vi "Image_Acquisition_Stop.vi"(11 "input cluster":T1={"L16 Linear Actuator"="ASRL6::INSTR", "XE 1000 Pump"="COM10", "Camera1"="cam2", "Camera2"="cam3", "Img_Capt"=TRUE, "Actuator"=TRUE, "Pump"=TRUE, "Cam 1"=TRUE, "Cam 2"=TRUE, "Empty_Refill"=FALSE, "Crop"=TRUE, "Light intensity"=50, "Exposure Time"=1000.0, "Sample Name"="Test Sample", "Operator"="MRJ", "Calibration 1"=path "C:/Users/au540322/Desktop/IHS_Project/calibration/Test Calibration/Test Calibration_7/1Test Calibration_7_2019_06_07-23-38-32-452.PNG", "Calibration 2"=path "C:/Users/au540322/Desktop/IHS_Project/calibration/Test Calibration/Test Calibration_7/2Test Calibration_7_2019_06_07-23-38-32-415.PNG", "Framerate"=1, "Timeout Sample"=50, "Collection date"="First test samples", "Sample size threshold"=1, "Empty start"=1, "Command"="MRJ", "Station"="", "Species Name"="", "Other Notes"="", "Aperture"=enum."Item 0", "Image Process Queue Size"=500, "Image Save Queue Size"=500, "Overload threshold"=500, "Max Framerate"=100, "Rectangle 1"={"Left"=0, "Top"=0, "Right"=0, "Bottom"=0, "Rotation"=0.0}, "Rectangle 2"={"Left"=0, "Top"=0, "Right"=0, "Bottom"=0, "Rotation"=0.0}, "Detection Region %"=0.0, "Detect 1"=path "C:/Users/au540322/Desktop/IHS_Project/images/Debris/Debris_0/Debris_0_2019_06_01-23-32-49-686.PNG", "Detect 2"=path "C:/Users/au540322/Desktop/IHS_Project/images/Debris/Debris_0/Debris_0_2019_06_01-23-32-49-686.PNG", "Max large object threshold"=0, "Open(T)/Close(F)"=FALSE, "Img_Capt Begin"=FALSE, "Dispense Speed"=100, "Flush Size"=100, "Location"="Station", "Latitude"="Station", "Longitude"="Station", "Determiner"="Station", "Sex"="Station", "Camera1_Img"="remote image 0000000015E6FBB4", "Camera2_Img"="remote image 0000000015E6F134", "Img1_Orig_Disp"=refnum, "Img2_Orig_Disp"=refnum, "Img1_Orig_RGB"=refnum, "Img2_Orig_RGB"=refnum, "Blue_Plane_Extract"=refnum, "Subtracted_Plane"=refnum, "Img1_Binary"=refnum, "Img2_Binary"=refnum, "Crop_Mask"=refnum, "Img1_Save"=refnum, "Img2_Save"=refnum, "Img1_Cali_Full"=refnum, "Img2_Cali_Full"=refnum, "Img1_Cali_Detect"=refnum, "Img2_Cali_Detect"=refnum, "Cam 1 queue"=refnum, "Cam 2 queue"=refnum, "Cam 1 - save queue"=refnum, "Cam 2 - save queue"=refnum} {"Flush Size" min=1; "Dispense Speed" min=1; "Rectangle 2"."Rotation" format="%.2f"; "Rectangle 2"."Left" scale=0.0..1024.0; "Rectangle 2"."Right" scale=0.0..1024.0; "Rectangle 1"."Rotation" format="%.2f"; "Rectangle 1"."Left" scale=0.0..1024.0; "Rectangle 1"."Right" scale=0.0..1024.0; "Max Framerate" min=1; "Overload threshold" min=1; "Image Save Queue Size" min=1; "Image Process Queue Size" min=1; "Empty start" min=1; "Sample size threshold" min=1; "Framerate" min=1; "Light intensity" scale=0.0..100.0}) -> (3 "output cluster":T1={"L16 Linear Actuator"="ASRL6::INSTR", "XE 1000 Pump"="COM10", "Camera1"="cam2", "Camera2"="cam3", "Img_Capt"=TRUE, "Actuator"=TRUE, "Pump"=TRUE, "Cam 1"=TRUE, "Cam 2"=TRUE, "Empty_Refill"=FALSE, "Crop"=TRUE, "Light intensity"=50, "Exposure Time"=1000.0, "Sample Name"="Test Sample", "Operator"="MRJ", "Calibration 1"=path "C:/Users/au540322/Desktop/IHS_Project/calibration/Test Calibration/Test Calibration_7/1Test Calibration_7_2019_06_07-23-38-32-452.PNG", "Calibration 2"=path "C:/Users/au540322/Desktop/IHS_Project/calibration/Test Calibration/Test Calibration_7/2Test Calibration_7_2019_06_07-23-38-32-415.PNG", "Framerate"=1, "Timeout Sample"=50, "Collection date"="First test samples", "Sample size threshold"=1, "Empty start"=1, "Command"="MRJ", "Station"="", "Species Name"="", "Other Notes"="", "Aperture"=enum."Item 0", "Image Process Queue Size"=500, "Image Save Queue Size"=500, "Overload threshold"=500, "Max Framerate"=100, "Rectangle 1"={"Left"=0, "Top"=0, "Right"=0, "Bottom"=0, "Rotation"=0.0}, "Rectangle 2"={"Left"=0, "Top"=0, "Right"=0, "Bottom"=0, "Rotation"=0.0}, "Detection Region %"=0.0, "Detect 1"=path "C:/Users/au540322/Desktop/IHS_Project/images/Debris/Debris_0/Debris_0_2019_06_01-23-32-49-686.PNG", "Detect 2"=path "C:/Users/au540322/Desktop/IHS_Project/images/Debris/Debris_0/Debris_0_2019_06_01-23-32-49-686.PNG", "Max large object threshold"=0, "Open(T)/Close(F)"=FALSE, "Img_Capt Begin"=FALSE, "Dispense Speed"=100, "Flush Size"=100, "Location"="Station", "Latitude"="Station", "Longitude"="Station", "Determiner"="Station", "Sex"="Station", "Camera1_Img"="remote image 0000000015E6FBB4", "Camera2_Img"="remote image 0000000015E6F134", "Img1_Orig_Disp"=refnum, "Img2_Orig_Disp"=refnum, "Img1_Orig_RGB"=refnum, "Img2_Orig_RGB"=refnum, "Blue_Plane_Extract"=refnum, "Subtracted_Plane"=refnum, "Img1_Binary"=refnum, "Img2_Binary"=refnum, "Crop_Mask"=refnum, "Img1_Save"=refnum, "Img2_Save"=refnum, "Img1_Cali_Full"=refnum, "Img2_Cali_Full"=refnum, "Img1_Cali_Detect"=refnum, "Img2_Cali_Detect"=refnum, "Cam 1 queue"=refnum, "Cam 2 queue"=refnum, "Cam 1 - save queue"=refnum, "Cam 2 - save queue"=refnum} {"Flush Size" min=1; "Dispense Speed" min=1; "Rectangle 2"."Rotation" format="%.2f"; "Rectangle 2"."Left" scale=0.0..1024.0; "Rectangle 2"."Right" scale=0.0..1024.0; "Rectangle 1"."Rotation" format="%.2f"; "Rectangle 1"."Left" scale=0.0..1024.0; "Rectangle 1"."Right" scale=0.0..1024.0; "Max Framerate" min=1; "Overload threshold" min=1; "Image Save Queue Size" min=1; "Image Process Queue Size" min=1; "Empty start" min=1; "Sample size threshold" min=1; "Framerate" min=1; "Light intensity" scale=0.0..100.0})   [LabVIEW 2020]
doc: "Stops acquisition of images from cameras."
uses:
  controls/Data.ctl
  <vilib>/userDefined/High Color/IMAQdx.ctl
  <vilib>/vision/Image Controls.llb/IMAQ Image.ctl
  <vilib>/vision/driver/NI_Vision_Acquisition_Software.lvlib
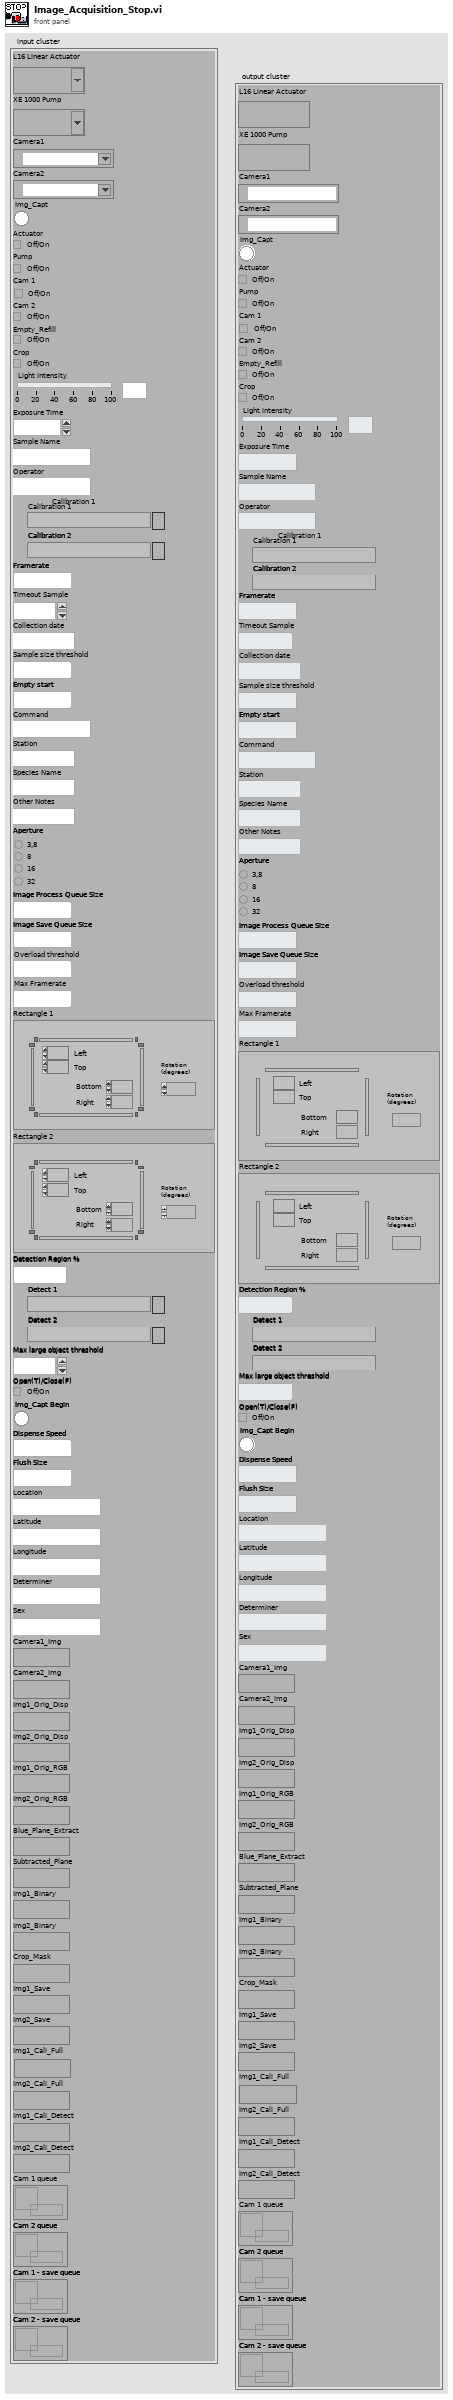
[diagram p1: front panel]
types:
  T1 = typedef "Data.ctl" = cluster{"L16 Linear Actuator":refnum<visa-resource-name>, "XE 1000 Pump":refnum<visa-resource-name>, "Camera1":T2, "Camera2":T2, "Img_Capt":bool, "Actuator":bool, "Pump":bool, "Cam 1":bool, "Cam 2":bool, "Empty_Refill":bool, "Crop":bool, "Light intensity":i32, "Exposure Time":dbl, "Sample Name":string, "Operator":string, "Calibration 1":path, "Calibration 2":path, "Framerate":i32, "Timeout Sample":i32, "Collection date":string, "Sample size threshold":i32, "Empty start":u32, "Command":string, "Station":string, "Species Name":string, "Other Notes":string, "Aperture":enum32{"Item 0", "Item 1", "Item 2", "Item 3"}, "Image Process Queue Size":i32, "Image Save Queue Size":i32, "Overload threshold":i32, "Max Framerate":i32, "Rectangle 1":T3, "Rectangle 2":T3, "Detection Region %":dbl, "Detect 1":path, "Detect 2":path, "Max large object threshold":i32, "Open(T)/Close(F)":bool, "Img_Capt Begin":bool, "Dispense Speed":i32, "Flush Size":i32, "Location":string, "Latitude":string, "Longitude":string, "Determiner":string, "Sex":string, "Camera1_Img":T4, "Camera2_Img":T4, "Img1_Orig_Disp":T4, "Img2_Orig_Disp":T4, "Img1_Orig_RGB":T4, "Img2_Orig_RGB":T4, "Blue_Plane_Extract":T4, "Subtracted_Plane":T4, "Img1_Binary":T4, "Img2_Binary":T4, "Crop_Mask":T4, "Img1_Save":T4, "Img2_Save":T4, "Img1_Cali_Full":T4, "Img2_Cali_Full":T4, "Img1_Cali_Detect":T4, "Img2_Cali_Detect":T4, "Cam 1 queue":refnum<queue>, "Cam 2 queue":refnum<queue>, "Cam 1 - save queue":refnum<queue>, "Cam 2 - save queue":refnum<queue>}
  T2 = typedef "IMAQdx.ctl" = refnum<k21>
  T3 = typedef "IMAQ Rectangle" = cluster{"Left":i32, "Top":i32, "Right":i32, "Bottom":i32, "Rotation":dbl}
  T4 = typedef "IMAQ Image.ctl" = refnum<image>
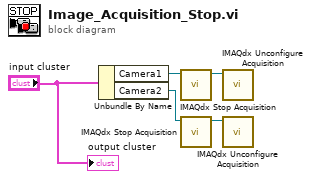
[diagram p0: block diagram]
diagram:
  n1 = Unbundle By Name("input cluster") -> ("Camera1"=w5:T2, "Camera2"=w3:T2)
  n2 = call <vilib>:"IMAQdx Stop Acquisition.vi"("Session In"=w5) -> ("Session Out"=w4:T2)  [unwired: 9 in, 1 out]
  n3 = call <vilib>:"IMAQdx Stop Acquisition.vi"("Session In"=w3) -> ("Session Out"=w2:T2)  [unwired: 9 in, 1 out]
  n4 = call <vilib>:"IMAQdx Unconfigure Acquisition.vi"("Session In"=w4) -> ()  [unwired: 9 in, 2 out]
  n5 = call <vilib>:"IMAQdx Unconfigure Acquisition.vi"("Session In"=w2) -> ()  [unwired: 9 in, 2 out]
  "output cluster" <- "input cluster"
